vi "Get Changed Data.vi"(0 "Serial port asssistant model in":refnum<class "Serial port assistant model.lvclass">, 11 "error in (no error)":errorcluster) -> (4 "Serial port asssistant model out":refnum<class "Serial port assistant model.lvclass">, 6 "view name":string, 8 "view number":i32, 10 "changed data":string, 15 "error out":errorcluster)   [LabVIEW 2022 SP3, in "Serial port assistant model.lvlib" / "Serial port assistant model.lvclass"]
uses:
  Serial port assistant model.lvclass
  Serial port assistant model.lvclass/Serial port assistant model.ctl
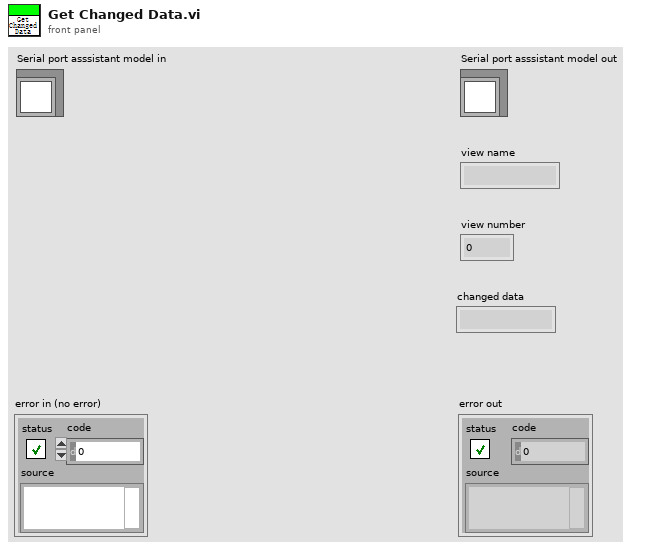
[diagram p1: front panel]
types:
  T1 = typedef "Serial port assistant model.lvlib/Serial port assistant model.lvclass/changed data--type.ctl" = cluster{"changed data":string}
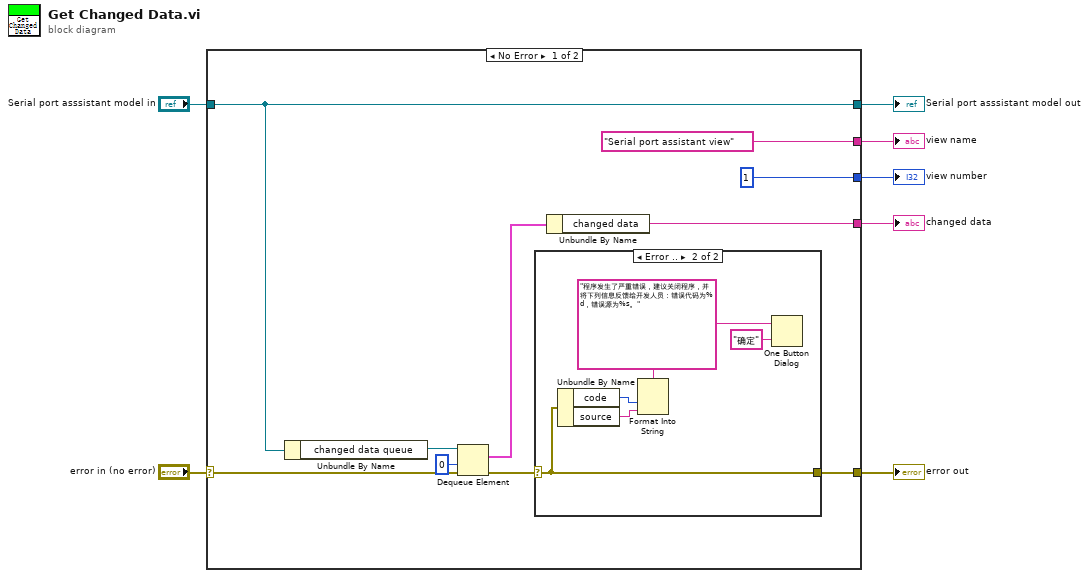
[diagram p0: block diagram]
diagram:
  n1 = case shown="No Error" "error in (no error)" {
    selector: "error in (no error)" -> [w17 w24]
    tunnel: "Serial port asssistant model in" -> [w16 w25]
    tunnel: [w16 w25] -> w5
    tunnel: [w8 w24] -> w4
    tunnel: [w10 _] -> w3
    tunnel: ["Serial port assistant view" _] -> w2
    tunnel: [1 _] -> w1
    frame No Error {
      n2 = Unbundle By Name(w16) -> ("changed data queue"=w15:refnum<queue>)
      n3 = Dequeue Element(queue=w15, timeout in ms (-1)=0, error in (no error)=w17) -> (element=w11:T1, error out=w9:errorcluster)  [unwired: 2 out]
      n4 = case shown="Error .." w9 {
        selector: w9 -> [w18 w19]
        tunnel: [w18 w19] -> w8
        frame No Error {
        }
        frame Error {
          w21 = "程序发生了严重错误，建议关闭程序，并将下列信息反馈给开发人员：错误代码为%d，错误源为%s。" ("format string")
          n5 = Unbundle By Name(w19) -> ("code"=w23:i32, "source"=w22:string)
          n6 = Format Into String(format string=w21, w23, w22) -> ()  [unwired: 2 in, 2 out]
          n7 = One Button Dialog(message=w21, button name ("OK")="确定") -> ()  [unwired: 1 out]
        }
      }
      n8 = Unbundle By Name(w11) -> ("changed data"=w10:string)
    }
    frame Error {
    }
  }
  "error out" <- w4
  "Serial port asssistant model out" <- w5
  "view name" <- w2
  "changed data" <- w3
  "view number" <- w1
